vi "module s Discover.vi"(7 "transport":i32, 8 "error in (no error)":errorcluster, 9 "stemListLength":i32, 10 "result":cluster{"value":i32, "error":i32}, 11 "id":u32) -> (0 "error out":errorcluster, 1 "stemListLength out":i32, 2 "result out":cluster{"value":i32, "error":i32}, 3 "id out":u32, 5 "stemList":u32[](array[numeric]))   [LabVIEW 2021, in "BrainStem2_LabVIEW_Library.lvlib"]
doc: "aLIBEXPORT void __stdcall module_sDiscover(\n unsigned int* id, \n struct Result* result, \n struct deviceListItem* stemList, \n int* stemListLength, \n int transport = (int)USB);"
uses:
  BrainStem2_LabVIEW_Library.lvlib
  BrainStem2_LabVIEW.dll
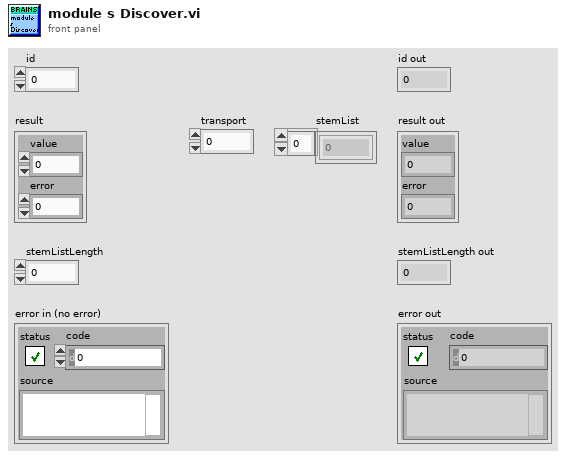
[diagram p1: front panel]
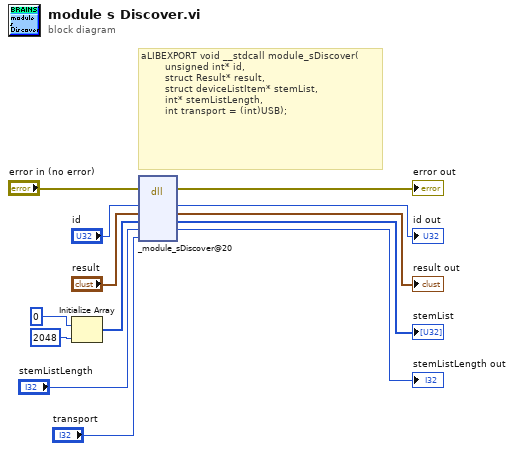
[diagram p0: block diagram]
diagram:
  # "aLIBEXPORT void __stdcall module_sDiscover(\n        unsigned int* id, \n        struct Result* result, \n        struct deviceListItem* stemList, \n        int* stemListLength, \n        int transport = (int)USB);"
  n1 = Initialize Array(u32 0 ("element"), 2048 ("dimension size")) -> (w9:u32[])
  n2 = dll-call lib="C:/DEV-TDS/Canary/T20029/T20029-80004 BS2 PROG SW/src/drivers/acroname/BrainStem2_LabVIEW.*" fn="_module_sDiscover@20"(error in="error in (no error)", "id"="id", "result"="result", "stemList"=w9, "stemListLength"="stemListLength", "transport"="transport") -> (error out=→"error out":errorcluster, "id"=→"id out":u32, "result"=→"result out":cluster{"value":i32, "error":i32}, "stemList"=→"stemList":u32[], "stemListLength"=→"stemListLength out":i32)  [unwired: 4 in, 1 out]
